vi "rx QPSK.vi"() -> ()   [LabVIEW 2026]
uses:
  <vilib>/addons/Modulation/niDMT.lvlib
  <vilib>/addons/Modulation/Digital/Demodulation/MT Calculate BER After Trigger (User Pattern).vi
  <instrlib>/niUSRP/niUSRP Fetch Rx Data (CDB Cluster).vi
panel:
  in  "path":path
  in  "device names":refnum<k15>
  in  "pulse shaping filter (none)":T1(ring)=enum."Raised Cosine"
  out "Constellation Graph":T2(graph)
  out "BER":dbl=1.0 format="%.4f"
  out "output bit stream":i8[](array[numeric])
  in  "carrier frequency":dbl=434000000.0 format="%#_6p"
  in  "Rx IQ rate":dbl=400000.0
  in  "number of samples":i64=16536
  in  "Stop":bool
  out "Waveform Graph":dbl[][](graph)
  out "error out":errorcluster
  out "coerced gain":dbl format="%#_6f"
  out "coerced carrier frequency":dbl=1000000000.0 format="%#_6p"
  out "coerced IQ rate":dbl=400000.0 format="%.6p"
  in  "active antenna":string="RX2"
  in  "rx gain":dbl=20.0 format="%#_6f"
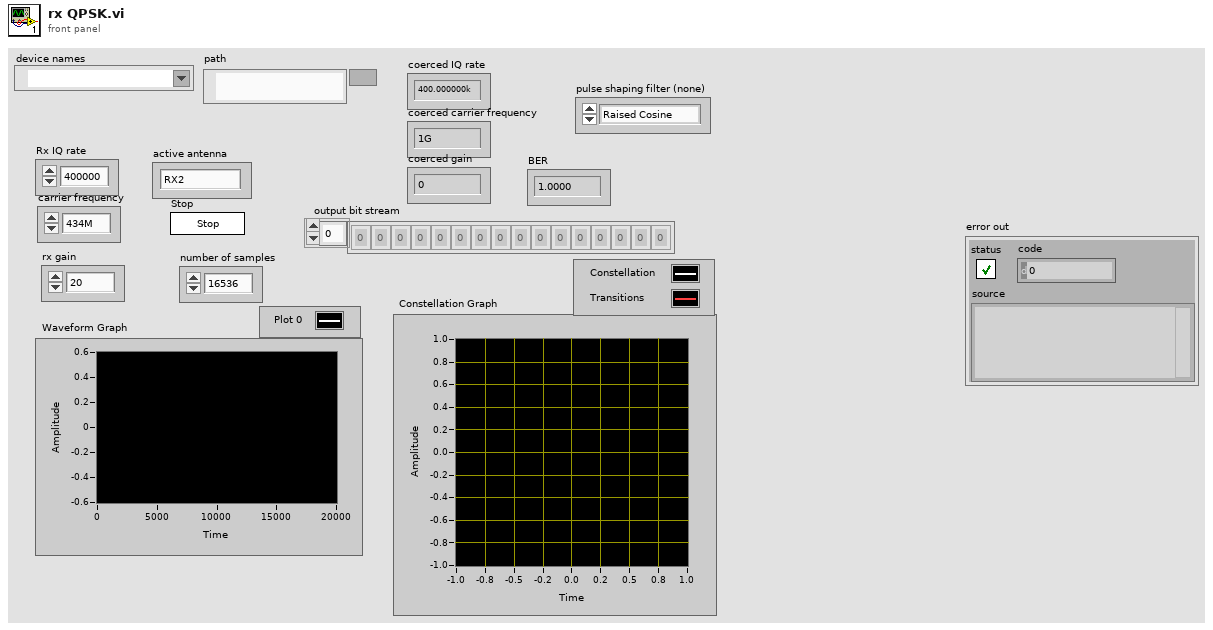
[diagram p1: front panel]
types:
  T1 = enum16{"none", "Raised Cosine", "Root Raised Cos", "Gaussian"}
  T2 = cluster{"constellation":dbl[], "oversampled data":dbl[]}[]
  T3 = cluster{"samples per symbol (16)":i32, "symbol map":cdb[], "differential PSK":enum16{"disable", "enable"}, "PSK type":u16}
  T4 = cluster{"expected sync location (symbols)":i32, "sync sequence":cdb[], "sync location uncertainty (symbols)":i32, "sync indent (symbols)":i32}
  T5 = typedef "niAMT.lvlib/Complex Data Waveform.ctl" = cluster{"t0":dbl, "dt":dbl, "Y":cdb[]}
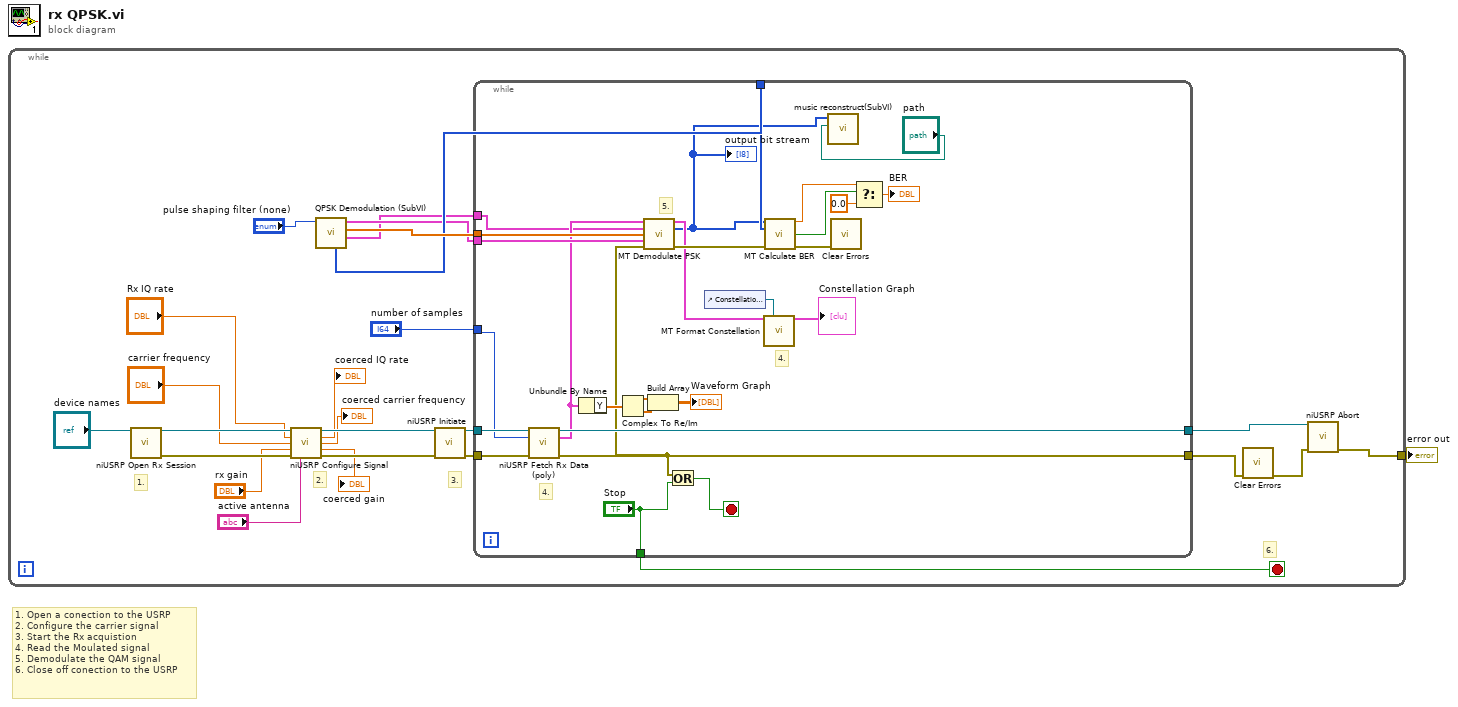
[diagram p0: block diagram]
diagram:
  # "1. Open a conection to the USRP\n2. Configure the carrier signal\n3. Start the Rx acquistion\n4. Read the Moulated signal\n5. Demodulate the QAM signal\n6. Close off conection to the USRP"
  n1 = while {
    tunnel: [w17] -> w1
    stop <- w8 stop-if-true
    # "6."
    # "3."
    # "2."
    # "1."
    n2 = call <instrlib>:"niUSRP Open Rx Session.vi"("device names"="device names") -> ("session handle out"=w26:refnum<k15>, "error out"=w25:errorcluster)  [unwired: 13 in]
    n3 = call <instrlib>:"niUSRP Configure Signal.vi"("session handle"=w26, "IQ rate"="Rx IQ rate", "carrier frequency"="carrier frequency", "gain"="rx gain", "error in (no error)"=w25, "active antenna"="active antenna") -> ("session handle out"=w21:refnum<k15>, "coerced IQ rate"=→"coerced IQ rate":dbl, "coerced carrier frequency"=→"coerced carrier frequency":dbl, "coerced gain"=→"coerced gain":dbl, "error out"=w22:errorcluster)  [unwired: 5 in]
    n4 = call "QPSK Demodulation (SubVI).vi"("pulse shaping filter (none)"="pulse shaping filter (none)") -> ("PSK system parameters"=w2:T3, "matched filter coefficients"=w7:dbl[], "QPSK synchronization parameters"=w3:T4, "output bit stream"=w6:i8[])  [unwired: 7 in]
    n5 = call <instrlib>:"niUSRP Initiate.vi"("session handle"=w21, "error in (no error)"=w22) -> ("session handle out"=w14:refnum<k15>, "error out"=w13:errorcluster)  [unwired: 12 in]
    n6 = while {
      tunnel: w14 -> [w53]
      tunnel: w13 -> [w52]
      tunnel: [w51] -> w12
      tunnel: [w41] -> w11
      tunnel: "number of samples" -> [w37]
      tunnel: ["Stop"] -> w8
      tunnel: w7 -> [w44]
      tunnel: w3 -> [w43]
      tunnel: w6 -> [w42]
      tunnel: w2 -> [w29]
      stop <- w47 stop-if-true
      # "4."
      # "4."
      # "5."
      n7 = call-poly <instrlib>:"niUSRP Fetch Rx Data (poly).vi"("session handle"=w53, "number of samples"=w37, "error in (no error)"=w52) -> ("session handle out"=w51:refnum<k15>, "data"=w34:cluster{"t0":dbl, "dt":dbl, "Y":cdb[]}, "error out"=w41:errorcluster)  [unwired: 9 in, 1 out]
      n8 = Unbundle By Name(w34) -> ("Y"=w45:cdb[])
      n9 = Complex To Re/Im(x + iy=w45) -> (x=w48:dbl[], y=w50:dbl[])
      n10 = call <vilib>:"MT Demodulate PSK.vi"("input complex waveform"=w34, "PSK system parameters"=w29, "matched filter coefficients"=w44, "synchronization parameters"=w43, "error in (no error)"=w41) -> ("recovered complex waveform"=w35:T5, "output bit stream"=w28:i8[], "error out"=w36:errorcluster)  [unwired: 6 in, 2 out]
      "output bit stream" <- w28
      n11 = Build Array(w48, w50) -> (→"Waveform Graph":dbl[][])
      n12 = Or(x=w41, y="Stop") -> (x .or. y?=w47:bool)
      n13 = control-ref of="Constellation Graph"() -> (w39:refnum<vi>)
      n14 = call <vilib>:"MT Format Constellation.vi"("waveform"=w35, "constellation reference"=w39) -> ("constellation graph"=→"Constellation Graph":T2)  [unwired: 3 in, 10 out]
      n15 = call-poly <vilib>:"MT Calculate BER.vi"("input bit stream"=w28, "reference bit pattern"=w42, "error in (no error)"=w36) -> ("BER"=w32:dbl, "trigger found?"=w33:bool, "error out"=w38:errorcluster)  [unwired: 8 in, 2 out]
      n16 = call "music reconstruct(SubVI).vi"("path"="path", "output bit stream in"=w28) -> ()  [unwired: 10 in]
      n17 = call <vilib>:"Clear Errors.vi"("error in (no error)"=w38) -> ()  [unwired: 5 in, 2 out]
      n18 = Select(t=w32, s=w33, f=0.0) -> (s? t:f=→"BER":dbl)
    }
    n19 = call <vilib>:"Clear Errors.vi"("error in (no error)"=w11) -> ("error out"=w9:errorcluster)  [unwired: 5 in, 1 out]
    n20 = call <instrlib>:"niUSRP Abort.vi"("session handle"=w12, "error in (no error)"=w9) -> ("error out"=w17:errorcluster)  [unwired: 12 in, 1 out]
  }
  "error out" <- w1
